vi "project.vi"() -> ()   [LabVIEW 2009]
panel:
  out "Boolean":bool
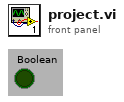
[diagram p1: front panel]
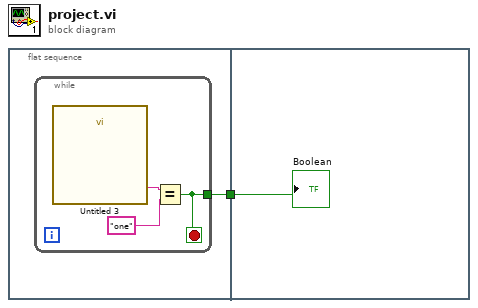
[diagram p0: block diagram]
diagram:
  n1 = flat-sequence {
    tunnel: [w2] -> w1
    tunnel: w1 -> [w6]
    frame #0 {
      n2 = while {
        tunnel: [w5] -> w2
        stop <- w5 stop-if-true
        n3 = call "Untitled 3.vi"() -> ("word"=w4:string)  [unwired: 17 in, 2 out]
        n4 = Equal?(x=w4, y="one") -> (x = y?=w5:bool)
      }
    }
    frame #1 {
      "Boolean" <- w6
    }
  }
